vi "Logging.vi"(7 "Name(\"\" to use uuid)":string="Logging") -> ()   [LabVIEW 2017, in "Logging.lvlib"]
uses:
  Logging.lvlib
  _support/Logging Configuration.ctl
  88f6bac4-2b4f-4fab-baa9-3cb27e3f7015.vi
  cb22bb73-ce69-4886-85ae-3a5aeb232168.vi
  d794aa55-fcc3-497b-8a77-67408dd3cb24.vi
  09a6c16d-484a-4fc5-8de7-d6b3640ac955.vi
  cc6353b5-7d2d-4e5e-85a1-4e3f7803f324.vi
  <userlib>/_NEVSTOP/Communicable State Machine(CSM)/AdvanceAPI/CSM - Revert Arguments-Safe String.vi
  <userlib>/_NEVSTOP/Communicable State Machine(CSM)/_Shared/Trim Single-line Text.vi
  <userlib>/_NEVSTOP/Communicable State Machine(CSM)/AdvanceAPI/CSM - Make String Arguments Safe.vi
  <userlib>/_NEVSTOP/Communicable State Machine(CSM)/AdvanceAPI/CSM - Break Down Multiple States String.vi
  <userlib>/_NEVSTOP/Communicable State Machine(CSM)/AdvanceAPI/CSM - Compact Multiple States.vi
  88f6bac4-2b4f-4fab-baa9-3cb27e3f7015.vi/99de0c97-112a-4c86-9094-c187659127e1.vi
  <userlib>/_NEVSTOP/Communicable State Machine(CSM)/Utility/Build Error Cluster.vi
  cb22bb73-ce69-4886-85ae-3a5aeb232168.vi/99de0c97-112a-4c86-9094-c187659127e1.vi
  <vilib>/Utility/error.llb/Clear Errors.vi
  <userlib>/_NEVSTOP/Communicable State Machine(CSM)/AdvanceAPI/CSM - Keywords.vi
  <vilib>/Utility/Data Type/Get Type Information.vi
  <userlib>/_NEVSTOP/Communicable State Machine(CSM)/addons/API-String-Arugments-Support/_Support/Data To SingleElementsArray_csm.vi
  <userlib>/_NEVSTOP/Communicable State Machine(CSM)/addons/API-String-Arugments-Support/_Support/Data To API String Arguments.vi
  <userlib>/_NEVSTOP/Communicable State Machine(CSM)/addons/INI-Static-Variable-Support/_Support/Parse Used Session and Name.vi
  <userlib>/_NEVSTOP/Communicable State Machine(CSM)/addons/INI-Static-Variable-Support/_Support/INI-FGV(lvlibp).vi
  <userlib>/_NEVSTOP/Communicable State Machine(CSM)/addons/INI-Static-Variable-Support/_Support/Populate String with INI Variable.vi
  <userlib>/_NEVSTOP/Communicable State Machine(CSM)/addons/API-String-Arugments-Support/_Support/Convert API String Arguments to Data(variant).vi
  <userlib>/_NEVSTOP/Communicable State Machine(CSM)/addons/API-String-Arugments-Support/_Support/SingleElementsArray To Data_csm.vi
  <userlib>/_NEVSTOP/Communicable State Machine(CSM)/addons/API-String-Arugments-Support/_Support/Query Data as API String Arguments(variant).vi
  <userlib>/_NEVSTOP/Communicable State Machine(CSM)/addons/MassData-Parameter/_support/FGV-MassData(lvlibp).vi
  <userlib>/_NEVSTOP/Communicable State Machine(CSM)/Communicable State Machine.lvlib
  <userlib>/_NEVSTOP/Communicable State Machine(CSM)/addons/Logger/CSM File Logger.lvlib
panel:
  out "Error Occurred":errorcluster
  out "State History":string
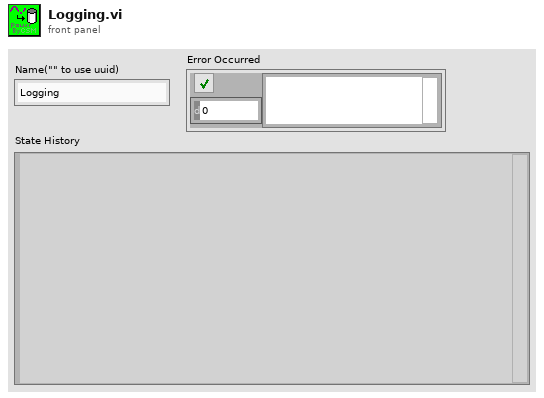
[diagram p1: front panel]
types:
  T1 = enum32{"Invalid", "Standard", "Closed", "Hidden", "Minimized", "Maximized"}
  T2 = enum32{"invalid app kind", "Development System", "Run Time System", "Student Edition", "Embedded LabVIEW", "Evaluation", "Custom"}
  T3 = enum16{"open", "open or create", "create or replace", "create", "open (read-only)"}
  T4 = typedef "Communicable State Machine.lvlib/_CSM_Response Source Message.ctl" = cluster{"‘State":string, "’Arguments":string, "’Error":errorcluster}
  T5 = cluster{"Current VI Reference":refnum<vi>, "Close Panel on Exit?":bool}
  T6 = typedef "Logging.lvlib/Logging Configuration.ctl" = cluster{"BasePath":path}
  T7 = cluster{"Core":cluster{"Current VI Reference":refnum<vi>, "Close Panel on Exit?":bool}, "Logging State":enum16{"Idle", "Logging"}, "tdms":refnum<k34>, "Configuration":T6}
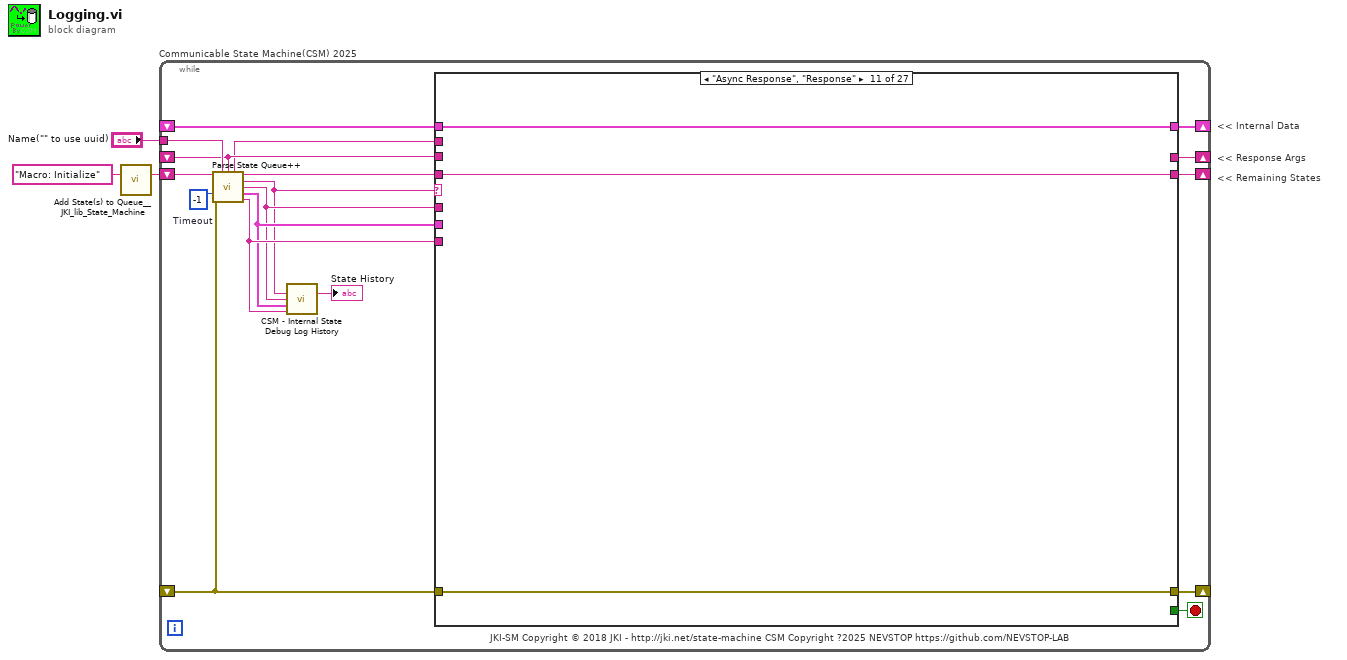
[diagram p0: block diagram]
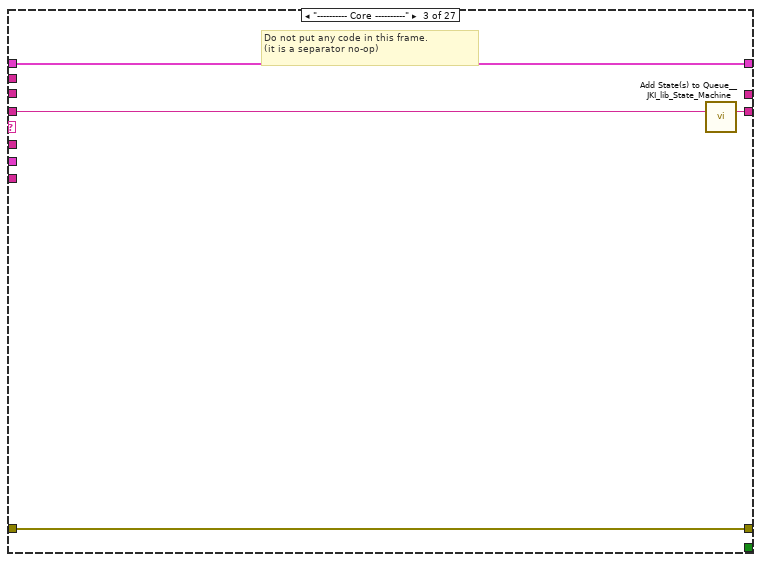
[diagram p4: hidden frame]
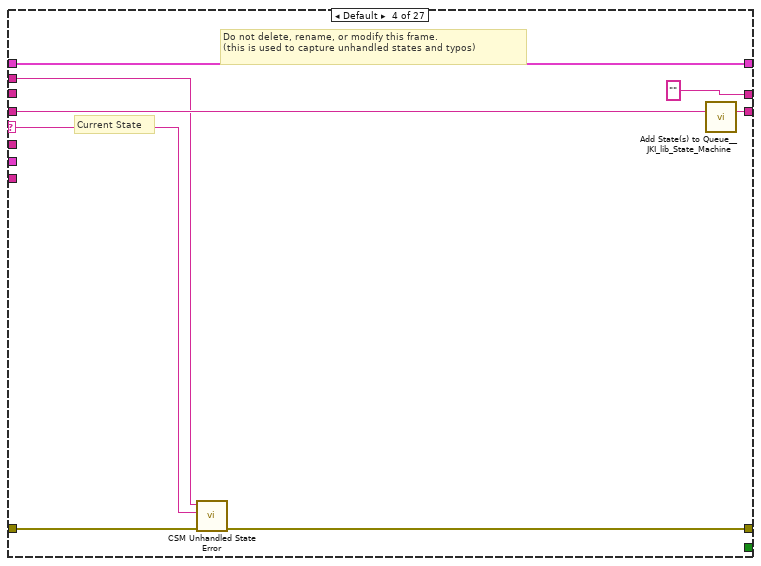
[diagram p5: hidden frame]
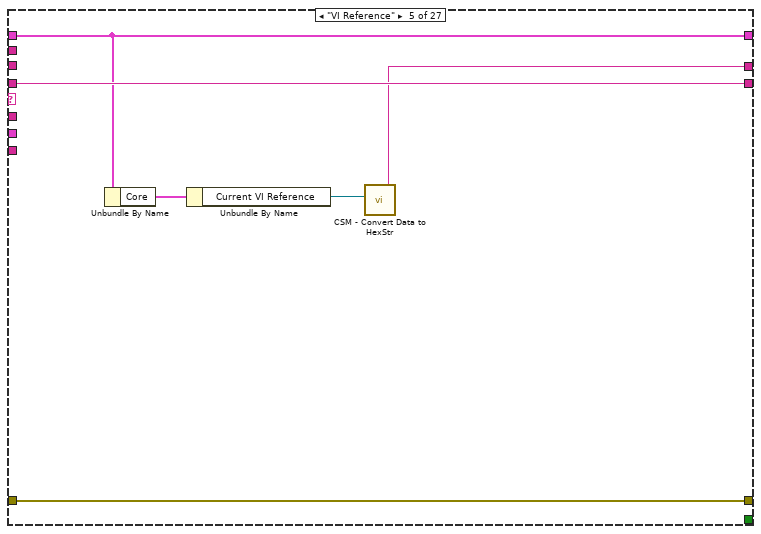
[diagram p6: hidden frame]
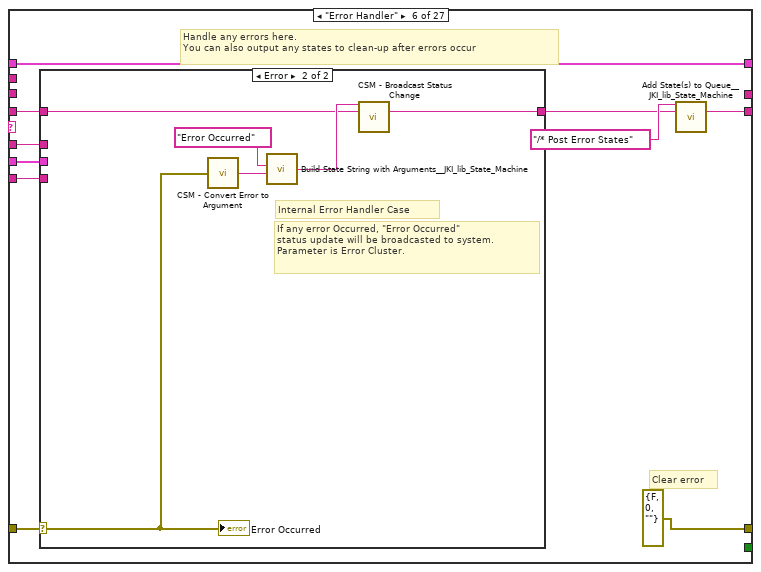
[diagram p7: hidden frame]
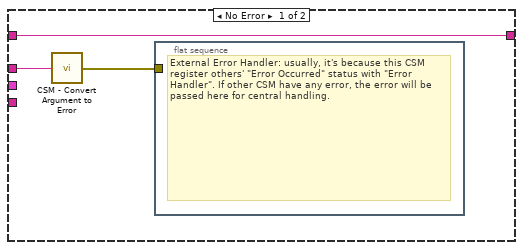
[diagram p8: hidden frame]
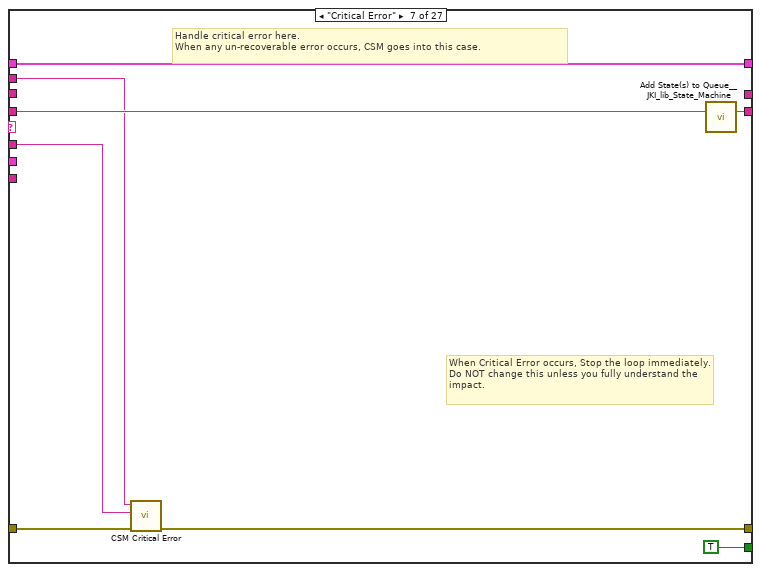
[diagram p9: hidden frame]
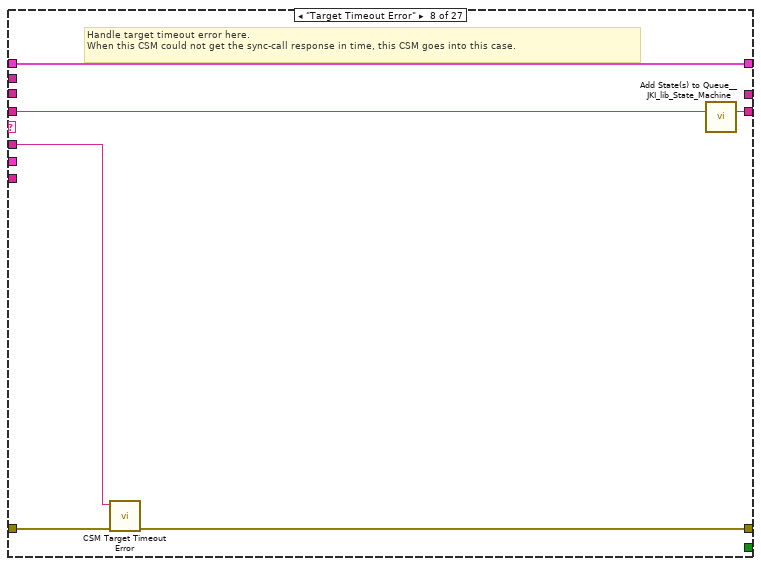
[diagram p10: hidden frame]
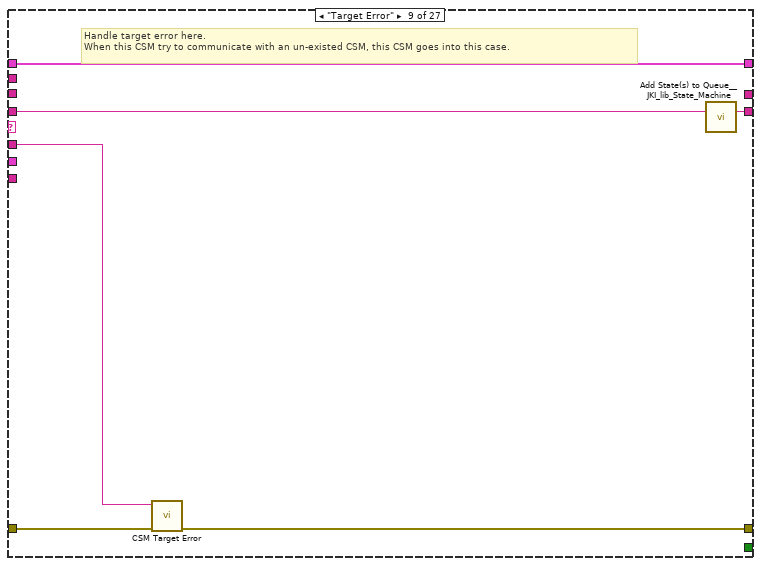
[diagram p11: hidden frame]
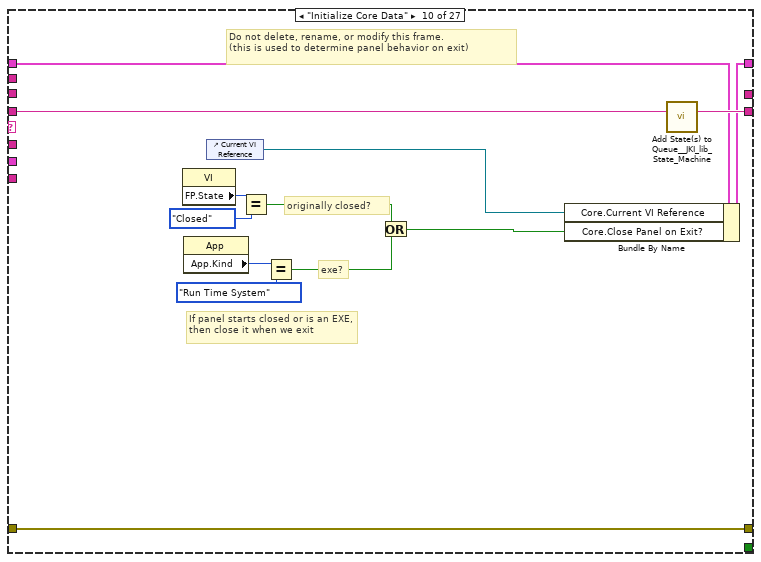
[diagram p12: hidden frame]
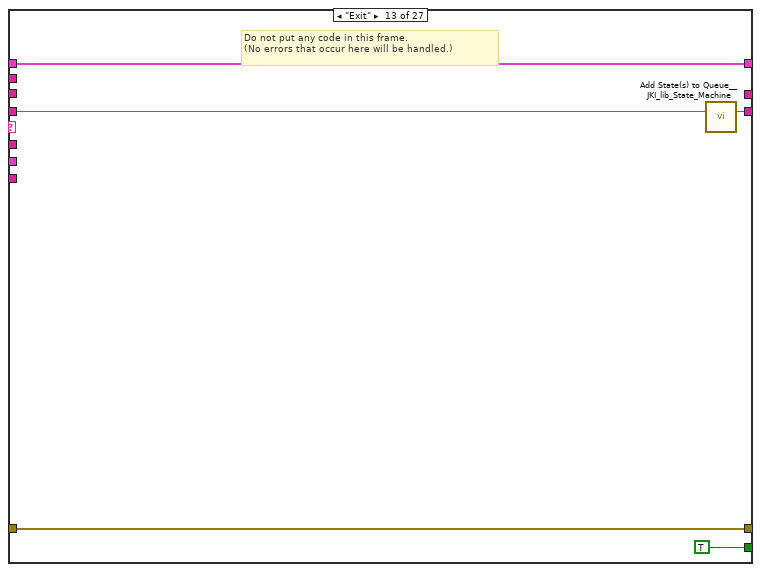
[diagram p14: hidden frame]
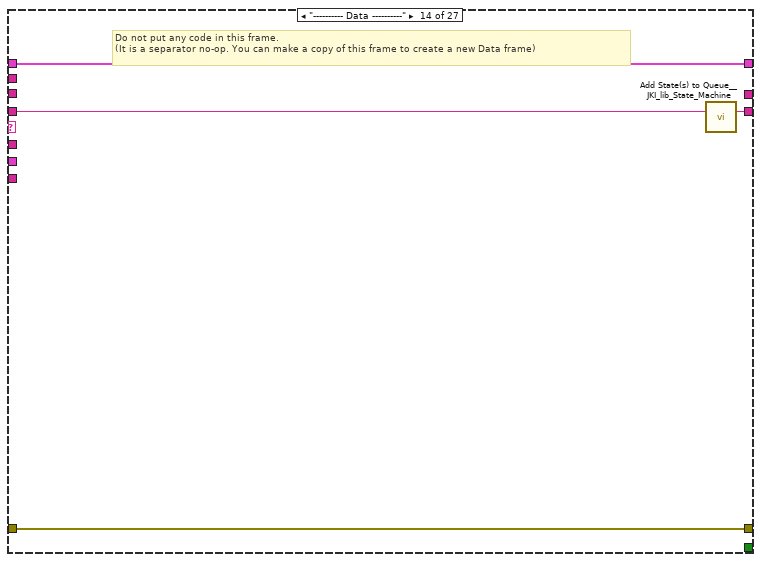
[diagram p15: hidden frame]
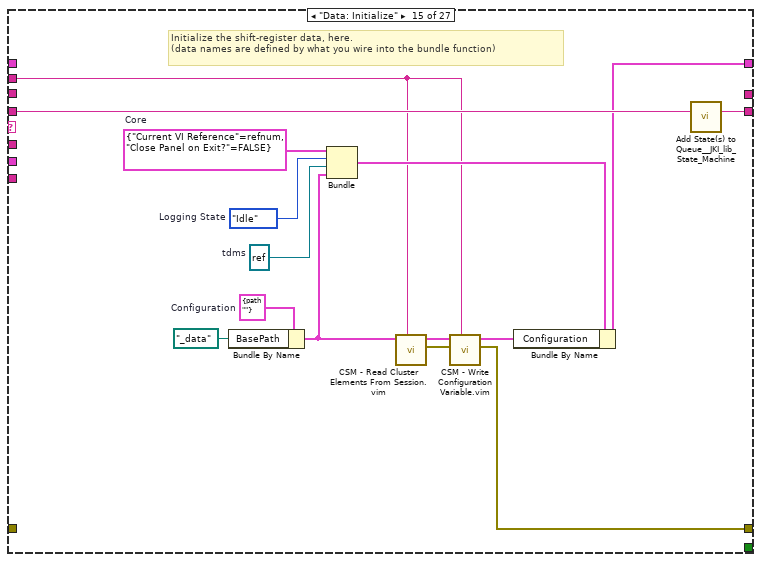
[diagram p16: hidden frame]
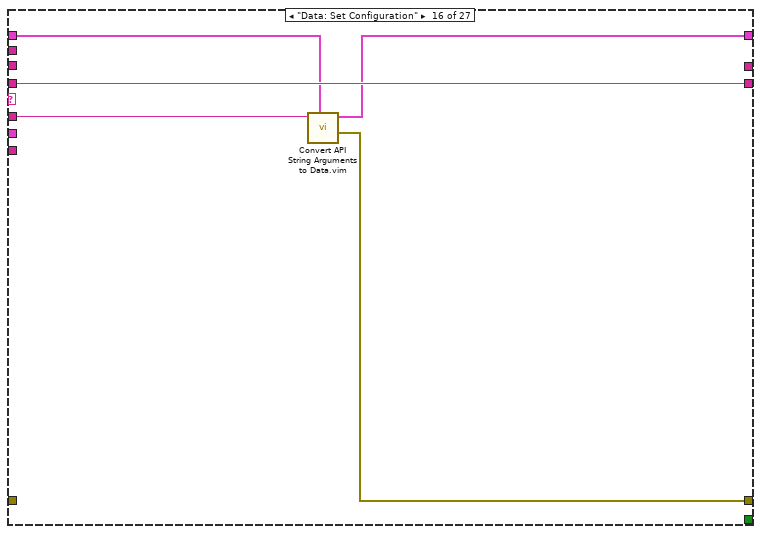
[diagram p17: hidden frame]
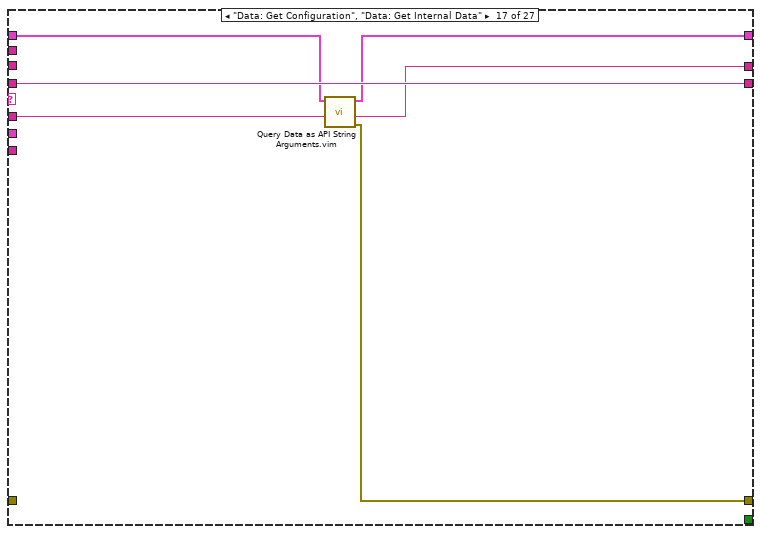
[diagram p18: hidden frame]
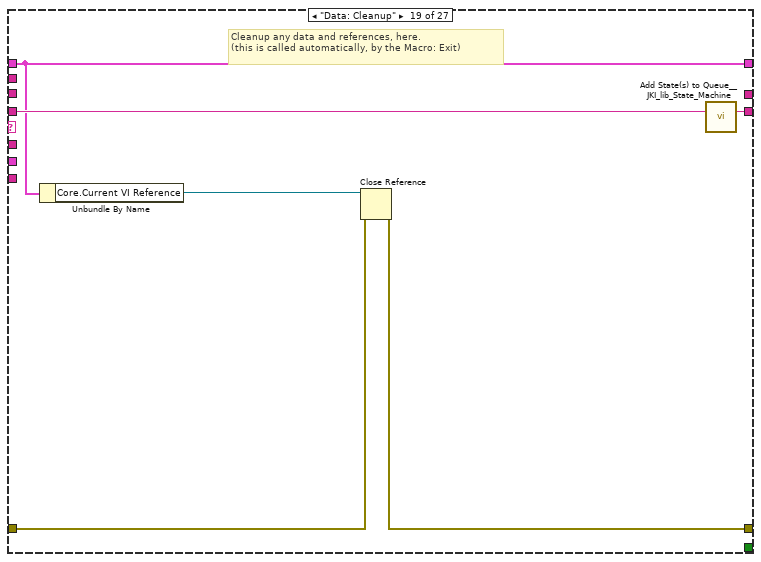
[diagram p20: hidden frame]
diagram:
  # "<< Internal Data"
  # "<< Response Args"
  # "<< Remaining States"
  n1 = call <vilib>:"Add State(s) to Queue__JKI_lib_State_Machine.vi"("State(s) in (\"\")"="Macro: Initialize") -> ("States Out"=w1:string)  [unwired: 14 in]
  n2 = while "Communicable State Machine(CSM) 2025" {
    shift-right: [w16] -> _
    shift-left: _ -> [w15]
    shift-right: [w19] -> _
    shift-left: _ -> [w14]
    shift-right: [w18] -> _
    shift-left: w1 -> [w20]
    tunnel: "Name(\"\" to use uuid)" -> [w11]
    shift-right: [w12] -> _
    shift-left: _ -> [w6]
    stop <- w17 stop-if-true
    w13 = -1  # Timeout
    # "JKI-SM Copyright © 2018 JKI - http://jki.net/state-machine CSM Copyright ?2025 NEVSTOP https://github.com/NEVSTOP-LAB"
    n3 = call <userlib>:"Parse State Queue++.vi"("State Queue"=w20, "Name (\"\" to Use UUID)"=w11, "Response Arguments"=w6, "Previous Error"=w14, "Dequeue (1 ms)"=w13) -> ("Name Used"=w5:string, "Remaining States"=w21:string, "Current State"=w7:string, "Arguments"=w8:string, "Additional Information"=w9:T4, "Source CSM"=w10:string)  [unwired: 5 in]
    n4 = call <userlib>:"CSM - Internal State Debug Log History.vi"("State"=w7, "Arguments (\"\")"=w8, ">> Response Source Message >>"=w9, "Source (\"\")"=w10) -> ("Debug Log"=→"State History":string)  [unwired: 11 in]
    n5 = case shown="\"Async Response\", \"Response\"" w7 {
      selector: w7 -> [_ _ _ w34 _ _ _ _ _ _ _ _ _ _ _ _ _ _ _ _ _ _ _ _ _ _ _]
      tunnel: w21 -> [w22 w26 w31 w38 w44 w49 w71 w77 w83 w97 w99 w102 w108 w112 w127 w132 w138 w140 w147 w151 w156 w161 w163 w172 w195 w210 w224]
      tunnel: w8 -> [_ _ _ _ _ w48 w67 w74 w80 _ _ _ _ _ _ w130 w135 _ _ _ _ _ _ _ w191 _ w221]
      tunnel: w15 -> [w23 w25 w28 w36 w43 w54 w69 w75 w81 w90 w98 w101 w106 w109 _ w131 w137 w139 w142 w148 w153 w158 w162 w170 w194 w208 w223]
      tunnel: [w24 w27 w29 w32 w45 errorcluster {"status"=FALSE, "code"=0, "source"=""} ("error out") w65 w73 w79 w94 w100 w103 w105 w110 w113 w129 w133 w141 w143 w149 w154 w159 w164 w168 w190 w205 w225] -> w19
      tunnel: w14 -> [w24 w27 w29 w39 w45 w52 w72 w78 w84 w94 w100 w103 w105 w110 _ _ _ w141 w144 w149 w154 w159 w164 _ w189 w206 w225]
      tunnel: [w22 w26 w30 w37 w44 w50 w70 w76 w82 w96 w99 w102 w107 w111 w126 w132 w138 w140 w146 w150 w155 w160 w163 w172 w195 w210 w224] -> w18
      tunnel: [_ _ _ _ _ _ TRUE _ _ _ _ _ TRUE _ _ _ _ _ _ _ _ _ _ _ _ _ _] -> w17
      tunnel: [w23 w25 w28 w36 w43 w54 w69 w75 w81 w95 w98 w101 w106 w109 w119 w128 w136 w139 w142 w148 w153 w158 w162 w169 w194 w207 w222] -> w16
      tunnel: w10 -> [_ _ _ _ _ w47 _ _ _ _ _ _ _ _ _ _ _ _ _ _ _ _ _ _ _ _ _]
      tunnel: w9 -> [_ _ _ _ _ w46 _ _ _ _ _ _ _ _ _ _ _ _ _ _ _ _ _ _ _ _ _]
      tunnel: [_ _ _ "" w40 _ _ _ _ _ _ _ _ _ _ _ w134 _ _ _ _ _ _ _ _ _ _] -> w12
      tunnel: w5 -> [_ _ _ w33 _ _ w66 _ _ _ _ _ _ _ w115 _ _ _ _ _ _ _ _ _ _ _ _]
      tunnel: w6 -> [_ _ _ _ _ _ _ _ _ _ _ _ _ _ _ _ _ _ _ _ _ _ _ _ _ _ _]
      frame "", "Idle" {
        # "README FIRST\n \nThis VI template should be used by dragging & dropping it from the Functions palette onto the Block Diagram of a new, blank VI, which will place it's contents into the blank VI. \nDo not edit the VI found in the palette.  Only edit the state machine after it is placed into your blank VI.\n \nFor instructions on how to use the JKI State Machine, examples and video tutorials, visit: http://jki.net/state-machine/\n\nJKI State Machine™\nhttp://jki.net/state-machine/\nCopyright (C) 2005-2018, JKI <info@jki.net>\nALL RIGHTS RESERVED\n\nFor information about CSM, visit: https://github.com/NEVSTOP-LAB"
        # "executes when the state queue is empty"
      }
      frame "CSM Documentation" {
        # "CSM Documentation"
        # "State Syntax:\nStateCategory: State >> Argument -@ CSMName\nStateCategory: State >> Argument -> CSMName\n\nLine Terminator: Line feed"
        # "Commenting:\nTo add a comment use \"//\" or \"#\" and all text to the right will be ignored\nCommenting Example:\nUI: Initialize // This initializes the UI\n// Another comment line"
        # "Example:\nUI: Help >> About -@Main\nUI: Help >> About ->Main\n\nWhere \"UI\" is the state category\nWhere \"Help\" is the state\nWhere \"About\" is the argument\nWhere \"Main\" is the Name of CSM,which actually run the \"UI: Help >> About\"\n\n    \"-@\" stands for sync state. Current CSM will wait until the state is finished. \n            - if \"Main\" named CSM does not exist, \"Target Error\" will occur.\n            - if \"Main\" named CSM is in another sync remote state, \"Target Busy Error\" will occur.\n            - if \"Main\" named CSM could not finish the state in time, \"Target Timeout Error\" will occur.\n            - if everything is right. \"Response\" will occur with Argument back from \"Main\" named CSM. \n\n    \"->\" stands for async state. Current CSM will post the state and continue to next state in next iteration.\n            - if \"Main\" named CSM does not exist, \"Target Error\" will occur.\n            - if everything is right. \"Async Message Posted\" will occur.\n            - After State is finished. Caller will receive a \"Async Response\" state from callee.\n\nWhen duplicated name is used for multiple CSM module or some framework problem happens, \"Critical Error\" will occur."
      }
      frame "---------- Core ----------" {
        # "Do not put any code in this frame.\n(it is a separator no-op)"
        n6 = call <vilib>:"Add State(s) to Queue__JKI_lib_State_Machine.vi"("State(s) in (\"\")"=w31) -> ("States Out"=w30:string)  [unwired: 14 in]
      }
      frame Default {
        # "Current State"
        # "Do not delete, rename, or modify this frame.\n(this is used to capture unhandled states and typos)"
        n7 = call <userlib>:"CSM Unhandled State Error.vi"("error in (no error)"=w39, "Undefined State"=w34, "CSM Name"=w33) -> ("error out"=w32:errorcluster)  [unwired: 8 in]
        n8 = call <vilib>:"Add State(s) to Queue__JKI_lib_State_Machine.vi"("State(s) in (\"\")"=w38) -> ("States Out"=w37:string)  [unwired: 14 in]
      }
      frame "VI Reference" {
        n9 = Unbundle By Name(w43) -> ("Core"=w42:T5)
        n10 = Unbundle By Name(w42) -> ("Current VI Reference"=w41:refnum<vi>)
        n11 = call <userlib>:"CSM - Convert Data to HexStr.vi"("Variant"=w41) -> ("HEX String (0-9,A-F)"=w40:string)  [unwired: 8 in]
      }
      frame "Error Handler" {
        # "Handle any errors here.\nYou can also output any states to clean-up after errors occur"
        # "Clear error"
        n12 = case shown="Error" w52 {
          selector: w52 -> [_ w59]
          tunnel: [w58 w61] -> w51
          tunnel: w49 -> [w58 w60]
          tunnel: w48 -> [w57 _]
          tunnel: w47 -> [_ _]
          tunnel: w46 -> [_ _]
          frame No Error {
            n13 = call <userlib>:"CSM - Convert Argument to Error.vi"("Argument"=w57) -> ("Error"=w56:errorcluster)  [unwired: 4 in]
            n14 = flat-sequence {
              tunnel: w56 -> [_]
              frame #0 {
                # "External Error Handler: usually, it's because this CSM register others' \"Error Occurred\" status with \"Error Handler\". If other CSM have any error, the error will be passed here for central handling."
              }
            }
          }
          frame Error {
            # "Internal Error Handler Case"
            # "If any error Occurred, \"Error Occurred\" \nstatus update will be broadcasted to system.\nParameter is Error Cluster."
            n15 = call <userlib>:"CSM - Convert Error to Argument.vi"("Error"=w59) -> ("Argument"=w63:string)  [unwired: 4 in]
            n16 = call <vilib>:"Build State String with Arguments__JKI_lib_State_Machine.vi"("Arguments (\"\")"=w63, "State"="Error Occurred" ("Status with Arguments")) -> ("State with Arguments"=w62:string)  [unwired: 4 in]
            n17 = call <userlib>:"CSM - Broadcast Status Change.vi"("Status With Arguments"=w62, "State Queue"=w60) -> ("Remaining States"=w61:string)  [unwired: 13 in]
            "Error Occurred" <- w59
          }
        }
        n18 = call <vilib>:"Add State(s) to Queue__JKI_lib_State_Machine.vi"("State(s) in Front (\"\")"="/* Post Error States", "State(s) in (\"\")"=w51) -> ("States Out"=w50:string)  [unwired: 13 in]
      }
      frame "Critical Error" {
        # "Handle critical error here.\nWhen any un-recoverable error occurs, CSM goes into this case."
        # "When Critical Error occurs, Stop the loop immediately. Do NOT change this unless you fully understand the impact."
        n19 = call <userlib>:"CSM Critical Error.vi"("error in (no error)"=w72, "Arugments (As Reason)"=w67, "CSM Name"=w66) -> ("error out"=w65:errorcluster)  [unwired: 8 in]
        n20 = call <vilib>:"Add State(s) to Queue__JKI_lib_State_Machine.vi"("State(s) in (\"\")"=w71) -> ("States Out"=w70:string)  [unwired: 14 in]
      }
      frame "Target Timeout Error" {
        # "Handle target timeout error here.\nWhen this CSM could not get the sync-call response in time, this CSM goes into this case."
        n21 = call <userlib>:"CSM Target Timeout Error.vi"("error in (no error)"=w78, "Arguments (As CSM Name)"=w74) -> ("error out"=w73:errorcluster)  [unwired: 9 in]
        n22 = call <vilib>:"Add State(s) to Queue__JKI_lib_State_Machine.vi"("State(s) in (\"\")"=w77) -> ("States Out"=w76:string)  [unwired: 14 in]
      }
      frame "Target Error" {
        # "Handle target error here.\nWhen this CSM try to communicate with an un-existed CSM, this CSM goes into this case."
        n23 = call <userlib>:"CSM Target Error.vi"("error in (no error)"=w84, "Arguments (As CSM Name)"=w80) -> ("error out"=w79:errorcluster)  [unwired: 9 in]
        n24 = call <vilib>:"Add State(s) to Queue__JKI_lib_State_Machine.vi"("State(s) in (\"\")"=w83) -> ("States Out"=w82:string)  [unwired: 14 in]
      }
      frame "Initialize Core Data" {
        # "Do not delete, rename, or modify this frame.\n(this is used to determine panel behavior on exit)"
        # "originally closed?"
        # "exe?"
        # "If panel starts closed or is an EXE, then close it when we exit"
        n25 = property class="VI"() -> ("FP.State"=w87:T1)  [unwired: 2 in, 2 out]
        n26 = property class="App"() -> ("App.Kind"=w93:T2)  [unwired: 2 in, 2 out]
        n27 = control-ref of="Current VI Reference"() -> (w88:refnum<vi>)
        n28 = Equal?(x=w87, y=T1."Closed" ("Front Panel Window:State")) -> (x = y?=w85:bool)
        n29 = Equal?(x=w93, y=T2."Run Time System" ("Application:Kind")) -> (x = y?=w91:bool)
        n30 = Or(x=w85, y=w91) -> (x .or. y?=w89:bool)
        n31 = Bundle By Name(cluster=w90, "Core.Current VI Reference"=w88, "Core.Close Panel on Exit?"=w89) -> (w95:T7)
        n32 = call <vilib>:"Add State(s) to Queue__JKI_lib_State_Machine.vi"("State(s) in (\"\")"=w97) -> ("States Out"=w96:string)  [unwired: 14 in]
      }
      frame "Async Response", "Response" {
      }
      frame "Async Message Posted" {
      }
      frame "Exit" {
        # "Do not put any code in this frame.\n(No errors that occur here will be handled.)"
        n33 = call <vilib>:"Add State(s) to Queue__JKI_lib_State_Machine.vi"("State(s) in (\"\")"=w108) -> ("States Out"=w107:string)  [unwired: 14 in]
      }
      frame "---------- Data ----------" {
        # "Do not put any code in this frame.\n(It is a separator no-op. You can make a copy of this frame to create a new Data frame)"
        n34 = call <vilib>:"Add State(s) to Queue__JKI_lib_State_Machine.vi"("State(s) in (\"\")"=w112) -> ("States Out"=w111:string)  [unwired: 14 in]
      }
      frame "Data: Initialize" {
        w121 = T6 {"BasePath"=path ""}  # Configuration
        w122 = refnum<k34> refnum  # tdms
        w123 = enum16{"Idle", "Logging"}."Idle"  # Logging State
        w124 = T5 {"Current VI Reference"=refnum, "Close Panel on Exit?"=FALSE}  # Core
        # "Initialize the shift-register data, here.\n(data names are defined by what you wire into the bundle function)"
        n35 = Bundle By Name(cluster=w121, "BasePath"=path "_data" ("name or relative path")) -> (w120:T6)
        n36 = Bundle("Core"=w124, "Logging State"=w123, "tdms"=w122, "Configuration"=w120) -> (w125:T7)  [unwired: 1 in]
        n37 = call "CSM - Read Cluster Elements From Session.vim"("Section Name (\"\" as Default)"=w115, "Cluster"=w120) -> ("error out"=w114:errorcluster, "Cluster out"=w118:T6)  [unwired: 6 in]
        n38 = call "CSM - Write Configuration Variable.vim"("Section Name (\"\" as Default)"=w115, "error in (no error)"=w114, "Configuration"=w118) -> ("error out"=w113:errorcluster, "Configuration (dup)"=w116:T6)  [unwired: 5 in]
        n39 = Bundle By Name(cluster=w125, "Configuration"=w116) -> (w119:T7)
        n40 = call <vilib>:"Add State(s) to Queue__JKI_lib_State_Machine.vi"("State(s) in (\"\")"=w127) -> ("States Out"=w126:string)  [unwired: 14 in]
      }
      frame "Data: Set Configuration" {
        n41 = call "Convert API String Arguments to Data.vim"("Reference Type"=w131, "API String"=w130) -> ("error out"=w129:errorcluster, "Data"=w128:T7)  [unwired: 6 in]
      }
      frame "Data: Get Configuration", "Data: Get Internal Data" {
        n42 = call "Query Data as API String Arguments.vim"("Name"=w135, "Cluster Data"=w137) -> ("error"=w133:errorcluster, "API String"=w134:string, "Cluster Data (dup)"=w136:T7)  [unwired: 7 in]
      }
      frame "Data: Update Indicators" {
      }
      frame "Data: Cleanup" {
        # "Cleanup any data and references, here.\n(this is called automatically, by the Macro: Exit)"
        n43 = Unbundle By Name(w142) -> ("Core.Current VI Reference"=w145:refnum<vi>)
        n44 = Close Reference(reference=w145, error in (no error)=w144) -> (error out=w143:errorcluster)
        n45 = call <vilib>:"Add State(s) to Queue__JKI_lib_State_Machine.vi"("State(s) in (\"\")"=w147) -> ("States Out"=w146:string)  [unwired: 14 in]
      }
      frame "---------- Macro ----------" {
        # "Do not put any code in this frame.\n(It is a separator no-op. You can make a copy of this frame to create a new Macro frame)"
        n46 = call <vilib>:"Add State(s) to Queue__JKI_lib_State_Machine.vi"("State(s) in (\"\")"=w151) -> ("States Out"=w150:string)  [unwired: 14 in]
      }
      frame "Macro: Initialize" {
        # "Initialization Macro\n(This is called once, when the VI starts)"
        n47 = call <vilib>:"Add State(s) to Queue__JKI_lib_State_Machine.vi"("State(s) in Front (\"\")"="Data: Initialize\nInitialize Core Data\nData: Update Indicators", "State(s) in (\"\")"=w156) -> ("States Out"=w155:string)  [unwired: 13 in]
      }
      frame "Macro: Exit" {
        # "Exit Macro\n(This is called once, when the VI exits)"
        n48 = call <vilib>:"Add State(s) to Queue__JKI_lib_State_Machine.vi"("State(s) in Front (\"\")"="Data: Cleanup\nExit", "State(s) in (\"\")"=w161) -> ("States Out"=w160:string)  [unwired: 13 in]
      }
      frame "---------- API ----------" {
        # "Do not put any code in this frame.\n(It is a separator no-op. This category is recommended to use for external API)"
      }
      frame "API: Start" {
        # "#CSM-NOTE\nto resolve relative path"
        # "Copy/Rename this case for your own API"
        n49 = Unbundle By Name(w170) -> ("Logging State"=w167:enum16{"Idle", "Logging"}, "Configuration.BasePath"=w166:path)
        n50 = call <userlib>:"Append CSM AppDir If Relative.vi"("Relative Path (.)"=w166) -> ("Application Directory (+ Relative)"=w165:path)  [unwired: 4 in]
        n51 = case shown="\"Idle\", Default" w167 {
          tunnel: w165 -> [w187 _]
          tunnel: "%Y_%m_%d_%H_%M_%S" -> [w186 _]
          tunnel: w170 -> [w177 w188]
          tunnel: [w176 w188] -> w169
          tunnel: [w174 _] -> w168
          frame "Idle", Default {
            n52 = call <vilib>:"Get File Extension.vi"("file"=w187) -> ("filename without extension"=w185:string, "lowercase file extension"=w182:string)  [unwired: 6 in, 3 out]
            n53 = Format Date/Time String(time format string (%c)=w186) -> (date/time string=w183:string)  [unwired: 2 in]
            n54 = call "__MGI Create Directory Chain.vi"("Path"=w187) -> ("Duplicate Path"=w173:path)  [unwired: 9 in, 1 out]
            n55 = Format Into String(format string="_%s.%s", initial string=w185, w183, w182) -> (resulting string=w181:string)  [unwired: 1 in, 1 out]
            n56 = Build Path(base path=w173, name or relative path=w181) -> (appended path=w180:path)
            n57 = TDMS Open(10:T3."create or replace" ("operation (0:open)"), 11:w180) -> (0:w174:errorcluster, 3:w178:refnum<k34>)  [unwired: 5 in]
            n58 = Bundle By Name(cluster=w177, "Logging State"=enum16{"Idle", "Logging"}."Logging", "tdms"=w178) -> (w176:T7)
          }
          frame "Logging" {
          }
        }
      }
      frame "API: Log" {
        n59 = Unbundle By Name(w194) -> ("Logging State"=w193:enum16{"Idle", "Logging"}, "tdms"=w192:refnum<k34>)
        n60 = case shown="\"Logging\"" w193 {
          tunnel: w192 -> [_ w203]
          tunnel: w191 -> [_ w201]
          tunnel: w189 -> [w196 w197]
          tunnel: [w196 w202] -> w190
          frame "Idle" {
            # "Ignore \"Log\" messages when the logging is idle."
          }
          frame "Logging" {
            # "Log more data while in the \"Logging\" state."
            n61 = call "CSM - Convert Argument to MassData.vim"("Type"=waveform(dbl)[] [] ("data"), "error in (no error)"=w197, "MassData Argument"=w201) -> ("error out"=w198:errorcluster, "Data"=w199:waveform(dbl)[])  [unwired: 5 in]
            n62 = TDMS Write(0:w203, 9:w199, 11:w198) -> (15:w202:errorcluster)  [unwired: 3 in, 3 out]
          }
        }
      }
      frame "API: Stop" {
        # "Copy/Rename this case for your own API"
        n63 = Unbundle By Name(w208) -> ("Logging State"=w204:enum16{"Idle", "Logging"}, "tdms"=w209:refnum<k34>)
        n64 = case shown="\"Logging\"" w204 {
          tunnel: w209 -> [_ w215]
          tunnel: w208 -> [w211 w219]
          tunnel: [w211 w218] -> w207
          tunnel: w206 -> [w212 w214]
          tunnel: [w212 w213] -> w205
          frame "Idle", Default {
          }
          frame "Logging" {
            n65 = TDMS Close(8:w214, 11:w215) -> (0:w213:errorcluster)  [unwired: 1 out]
            n66 = Bundle By Name(cluster=w219, "Logging State"=enum16{"Idle", "Logging"}."Idle", "tdms"=refnum<k34> refnum) -> (w218:T7)
          }
        }
      }
      frame "API: Update Settings" {
        # "Copy/Rename this case for your own API"
        n67 = String To Path(string=w221) -> (path=w220:path)
        n68 = Bundle By Name(cluster=w223, "Configuration.BasePath"=w220) -> (w222:T7)
      }
    }
  }
